vi "index_ctl.vi"(8 "错误输入（无错误）":errorcluster, 10 "lable":string, 11 "VI refence":refnum<vi>) -> (0 "error out":errorcluster, 3 "Ctl refence":refnum<vi>)   [LabVIEW 2013]
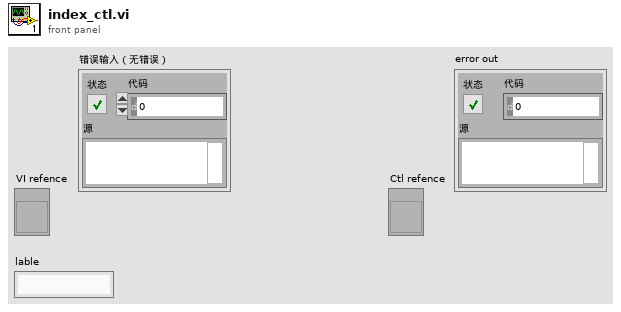
[diagram p1: front panel]
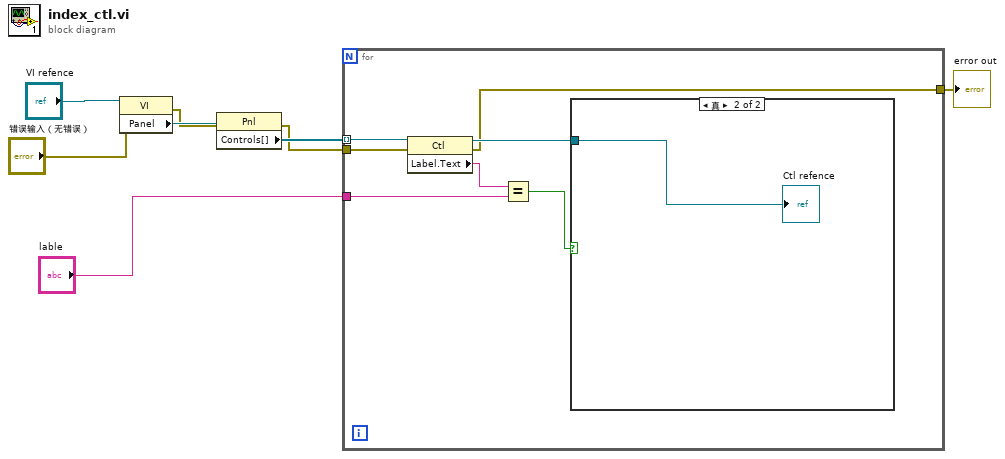
[diagram p0: block diagram]
diagram:
  n1 = property class="VI"(reference="VI refence", error in="错误输入（无错误）") -> (error out=w3:errorcluster, "Panel"=w8:refnum<vi>)  [unwired: 1 out]
  n2 = property class="Pnl"(reference=w8, error in=w3) -> (error out=w2:errorcluster, "Controls[]"=w7:refnum<vi>[])  [unwired: 1 out]
  n3 = for {
    tunnel: w7 -> [w15] mode=indexing
    tunnel: "lable" -> [w13]
    tunnel: w2 -> [w10]
    tunnel: [w9] -> w1
    n4 = property class="Ctl"(reference=w15, error in=w10) -> (reference out=w11:refnum<vi>, error out=w9:errorcluster, "Label.Text"=w14:string)
    n5 = Equal?(x=w14, y=w13) -> (x = y?=w12:bool)
    n6 = case shown="真" w12 {
      tunnel: w11 -> [_ w16]
      frame False {
      }
      frame True {
        "Ctl refence" <- w16
      }
    }
  }
  "error out" <- w1
